vi "SupplySwitch.vi"(8 "error in (no error)":errorcluster caption="错误输入（无错误）", 9 "Output":bool=TRUE, 10 "CH":enum16{"Positive", "Negative"}(ring), 11 "handle":u64) -> (0 "error out":errorcluster caption="错误输出", 2 "function return":i32, 3 "handle out":u64)   [LabVIEW 2018]
doc: "Open or Close Power Supply"
uses:
  InstrumentsPlayground.lvlib
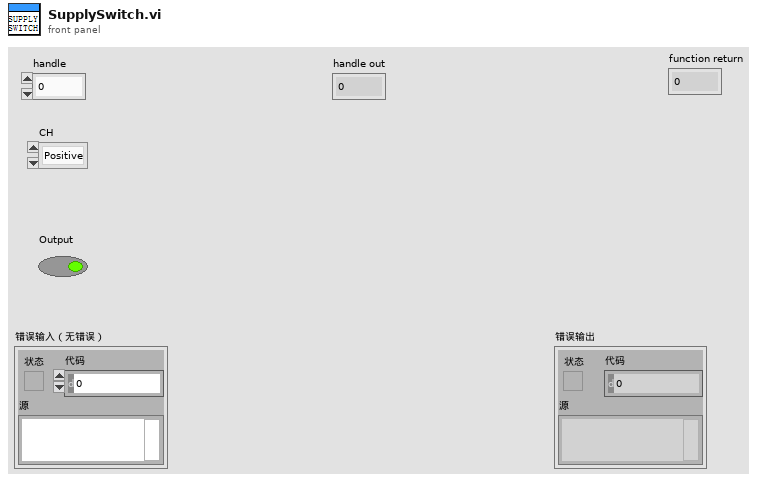
[diagram p1: front panel]
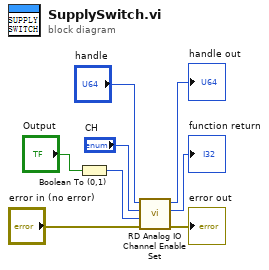
[diagram p0: block diagram]
diagram:
  n1 = Boolean To (0,1)(Boolean="Output") -> (0, 1=w1:i16)
  n2 = call "RD Analog IO Channel Enable Set.vi"("error in (no error)"="error in (no error)", "enable"=w1, "ch"="CH", "handle"="handle") -> ("error out"=→"error out":errorcluster, "function return"=→"function return":i32, "handle out"=→"handle out":u64)  [unwired: 5 in]
